vi "Begin.vi"() -> (1 "Темп-ра":dbl, 2 "№ об-ца":dbl, 3 "String":string)   [LabVIEW 2018]
panel:
  in  "№ образца:":dbl
  in  "Температура:":dbl
  in  "ОК (ОЗ)":bool
  in  "ОА(ОП)":bool
  out "Лампа":bool=TRUE
  # "Тип индикатора:"
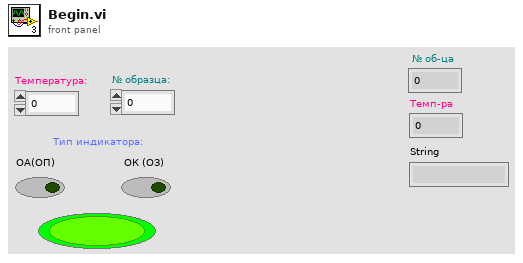
[diagram p1: front panel]
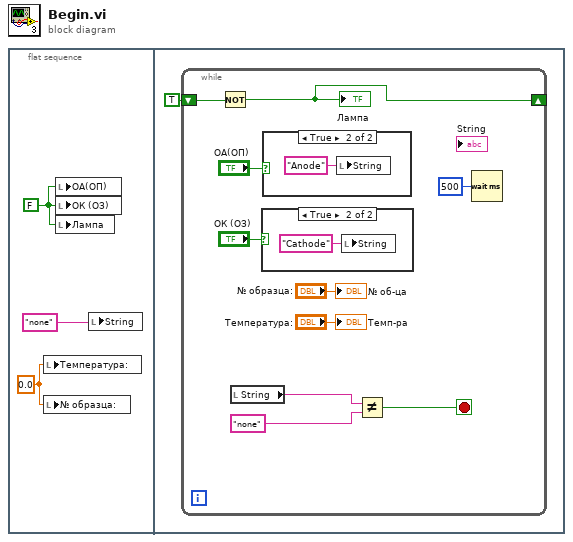
[diagram p0: block diagram]
diagram:
  n1 = flat-sequence {
    frame #0 {
      w1 = 0.0 ("Температура:")
      w3 = FALSE ("ОА (ОП)")
      n2 = local write "Температура:"(w1) -> ()
      n3 = local write "№ образца:"(w1) -> ()
      n4 = local write "ОА(ОП)"(w3) -> ()
      n5 = local write "ОК (ОЗ)"(w3) -> ()
      n6 = local write "Лампа"(w3) -> ()
      n7 = local write "String"("none" ("String")) -> ()
    }
    frame #1 {
      n8 = while {
        shift-right: [w12] -> _
        shift-left: TRUE -> [w13]
        stop <- w5 stop-if-true
        n9 = Not(x=w13) -> (.not. x?=w12:bool)
        "Лампа" <- w12
        n10 = local read "String"() -> (w11:string)
        n11 = case shown="True" "ОК (ОЗ)" {
          frame False {
          }
          frame True {
            n12 = local write "String"("Cathode" ("String")) -> ()
          }
        }
        n13 = case shown="True" "ОА(ОП)" {
          frame False {
          }
          frame True {
            n14 = local write "String"("Anode" ("String")) -> ()
          }
        }
        n15 = Not Equal?(x=w11, y="none") -> (x != y?=w5:bool)
        n16 = Wait (ms)(milliseconds to wait=u32 500) -> ()  [unwired: 1 out]
        "№ об-ца" <- "№ образца:"
        "Темп-ра" <- "Температура:"
      }
    }
  }
